vi "ma_Bilinear Prewarping of f.vi"(1 "f":dbl format="%0.2f") -> (0 "prewarped f":dbl format="%0.2f")   [LabVIEW 2020, in "NI_MAPro.lvlib"]
uses:
  NI_MAPro.lvlib
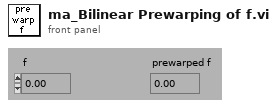
[diagram p1: front panel]
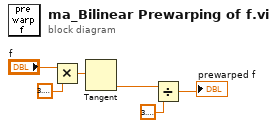
[diagram p0: block diagram]
diagram:
  n1 = Multiply(x="f", y=3.141592653589793) -> (x*y=w5:dbl)
  n2 = Tangent(1:w5) -> (0:w2:dbl)
  n3 = Divide(x=w2, y=3.141592653589793) -> (x/y=→"prewarped f":dbl)
